vi "Get MFC Gase.vi"(8 "Fehler (Eingang, kein Fehler)":errorcluster, 11 "mfc Gasnamen in":string[](array[string])) -> (0 "Fehler (Ausgang)":errorcluster)   [LabVIEW 2020, in "Linearisierung v2.lvlib" / "Gasteiler.lvlib" / "HovaCAL_Interface.lvlib" / "Kommunikation.lvlib"]
uses:
  Kommunikation.lvlib
  Aktion_FGV_HovaCAL_Interface_Gasliste.ctl
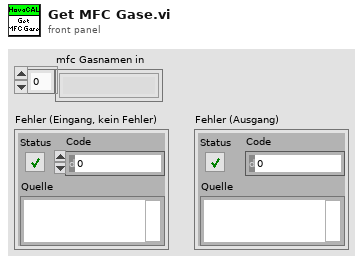
[diagram p1: front panel]
types:
  T1 = typedef "Linearisierung v2.lvlib/Gasteiler.lvlib/HovaCAL_Interface.lvlib/Kommunikation.lvlib/Aktion_FGV_HovaCAL_Interface_Gasliste.ctl" = enum16{"lesen", "setzen", "erstellen"}
  T2 = cluster{"HovaCAL Limits Cluster":refnum<vi>, "HovaCAL SetPumpMode":refnum<vi>, "HovaCAL Cluster.PumpModeGeneral":refnum<vi>, "HovaCAL SetPumpMode-Cluster":refnum<vi>, "HovaCAL Flow Input Cluster":refnum<vi>, "HovaCAL Set Values Cluster":refnum<vi>[], "HovaCAL Temperature":refnum<vi>, "HovaCAL Pump Concentrations-Cluster":refnum<vi>[], "HovaCAL AutoLin MFC":refnum<vi>, "HovaCAL MFC Gase Cluster Array out":refnum<vi>[]}
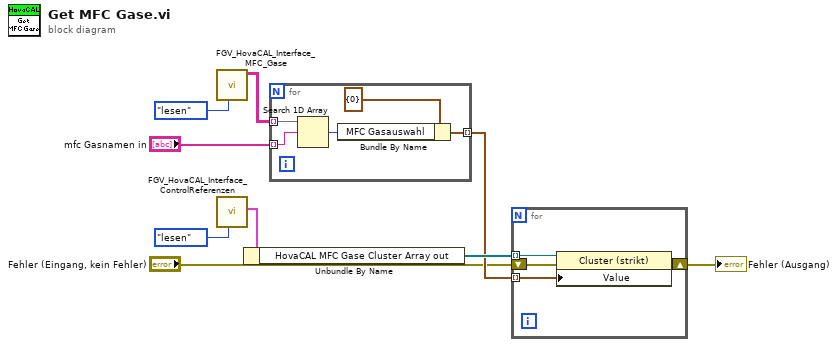
[diagram p0: block diagram]
diagram:
  n1 = call "FGV_HovaCAL_Interface_MFC_Gase.vi"("Aktion"=Aktion_FGV_HovaCAL_Interface_Gasliste."lesen") -> ("mfc Gaslisten out"=w5:string[][])  [unwired: 8 in, 2 out]
  n2 = call "FGV_HovaCAL_Interface_ControlReferenzen.vi"("Aktion"=enum16{"lesen", "schreiben"}."lesen") -> ("Set Cluster out"=w8:T2)  [unwired: 6 in, 4 out]
  n3 = Unbundle By Name(w8) -> ("HovaCAL MFC Gase Cluster Array out"=w6:refnum<vi>[])
  n4 = for {
    tunnel: w5 -> [w14] mode=indexing
    tunnel: "mfc Gasnamen in" -> [w13] mode=indexing
    tunnel: [w10] -> w3 mode=indexing
    n5 = Search 1D Array(1D array=w14, element=w13) -> (index of element=w11:i32)  [unwired: 1 in]
    n6 = Bundle By Name(cluster=cluster{"MFC Gasauswahl":u16} {"MFC Gasauswahl"=0} ("Wert"), "MFC Gasauswahl"=w11) -> (w10:cluster{"MFC Gasauswahl":u16})
  }
  n7 = for {
    tunnel: w6 -> [w18] mode=indexing
    tunnel: w3 -> [w17] mode=indexing
    shift-right: [w15] -> w1
    shift-left: "Fehler (Eingang, kein Fehler)" -> [w16]
    n8 = property class="Cluster (strikt)"(reference=w18, error in=w16, "Value"=w17) -> (error out=w15:errorcluster)  [unwired: 1 out]
  }
  "Fehler (Ausgang)" <- w1
